vi "open temporary ds opc.vi"(4 "read=f,write=t":bool, 6 "PLC Path and Tag in":T1 {"DataSocket Reference"."OnStatusUpdated" format="%.0x"; "DataSocket Reference"."OnDataUpdated" format="%.0x"}, 8 "error in":errorcluster, 9 "PLC/OPC Path":string, 10 "use opc":bool, 11 "PLC boolean read Tags":T1[](array[typedef]) {"DataSocket Reference"."OnStatusUpdated" format="%.0x"; "DataSocket Reference"."OnDataUpdated" format="%.0x"}) -> (0 "error out":errorcluster, 2 "close ds after io":bool, 3 "PLC Path and Tag out":T1 {"DataSocket Reference"."OnStatusUpdated" format="%.0x"; "DataSocket Reference"."OnDataUpdated" format="%.0x"})   [LabVIEW 2018]
uses:
  05.UserVI's/type defs/plc path and tag.ctl
  <vilib>/Platform/dataskt.llb/DataSocket Reference Type.ctl
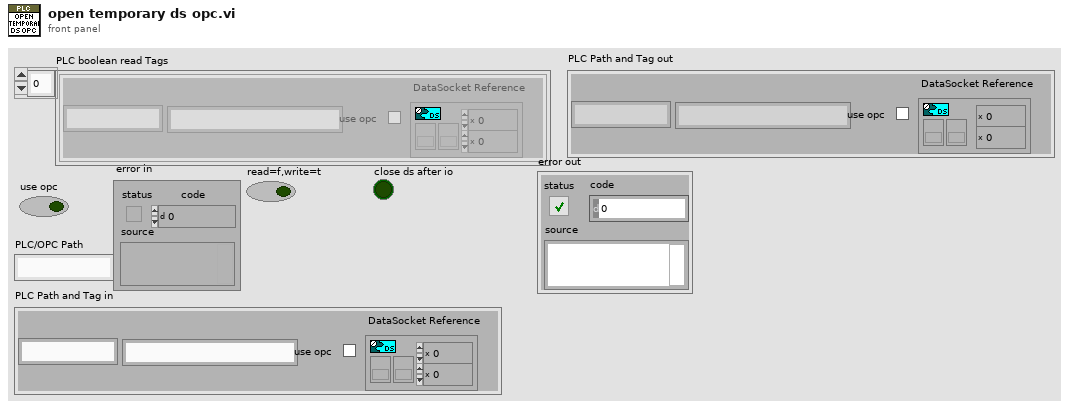
[diagram p1: front panel]
types:
  T1 = typedef "plc path and tag.ctl" = cluster{"Tag Name":string, "Network Path":string, "use opc":bool, "DataSocket Reference":T2}
  T2 = typedef "DataSocket Reference Type.ctl" = cluster{"CWDSLib._DCWDataSocket":refnum<k7>, "CWDSLib._DCWData":refnum<k7>, "OnDataUpdated":u32, "OnStatusUpdated":u32}
  T3 = enum32{"Reserved1", "Reserved2", "Read", "ReadAutoUpdate", "Write", "WriteAutoUpdate"}
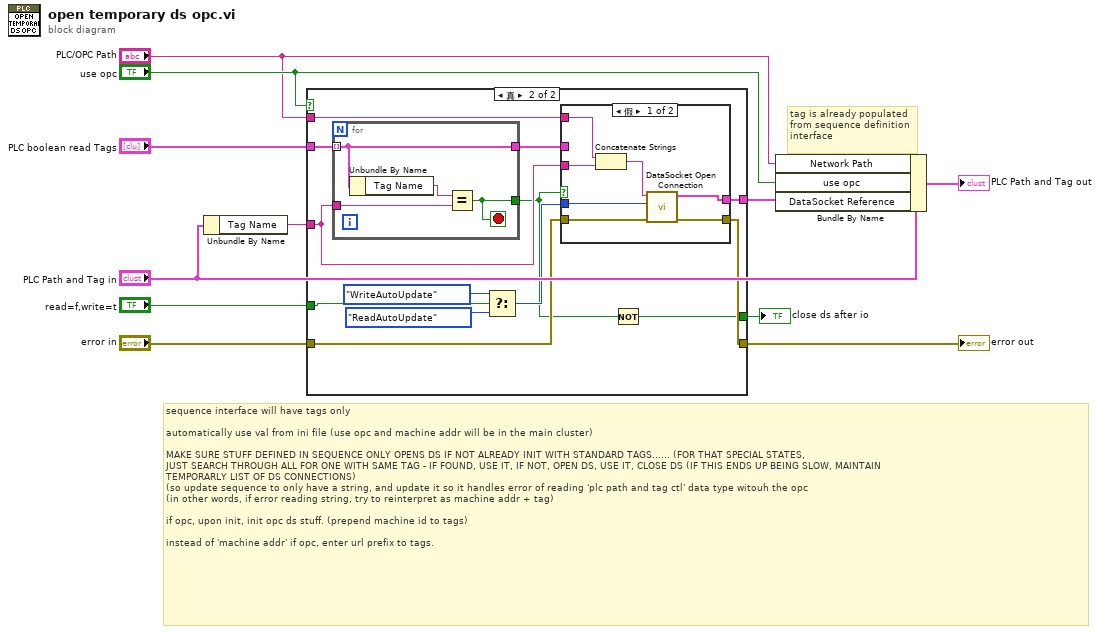
[diagram p0: block diagram]
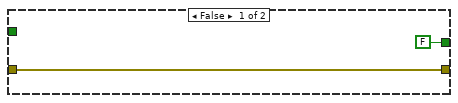
[diagram p2: hidden frame]
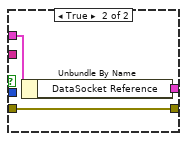
[diagram p3: hidden frame]
diagram:
  # "sequence interface will have tags only\n\nautomatically use val from ini file (use opc and machine addr will be in the main cluster) \n\nMAKE SURE STUFF DEFINED IN SEQUENCE ONLY OPENS DS IF NOT ALREADY INIT WITH STANDARD TAGS...... (FOR THAT SPECIAL STATES,\nJUST SEARCH THROUGH ALL FOR ONE WITH SAME TAG - IF FOUND, USE IT, IF NOT, OPEN DS, USE IT, CLOSE DS (IF THIS ENDS UP BEING SLOW, MAINTAIN\nTEMPORARLY LIST OF DS CONNECTIONS)\n(so update sequence to only have a string, and update it so it handles error of reading 'plc path and tag ctl' data type witouh the opc\n(in other words, if error reading string, try to reinterpret as machine addr + tag)\n\nif opc, upon init, init opc ds stuff. (prepend machine id to tags)\n\ninstead of 'machine addr' if opc, enter url prefix to tags."
  # "tag is already populated from sequence definition interface"
  n1 = Unbundle By Name("PLC Path and Tag in") -> ("Tag Name"=w11:string)
  n2 = case shown="真" "use opc" {
    tunnel: [_ w24] -> w8
    tunnel: "PLC boolean read Tags" -> [_ w26]
    tunnel: w11 -> [_ w20]
    tunnel: "error in" -> [w13 w23]
    tunnel: [w13 w22] -> w4
    tunnel: "PLC/OPC Path" -> [_ w21]
    tunnel: "read=f,write=t" -> [_ w19]
    tunnel: [FALSE w14] -> w1
    frame False {
    }
    frame True {
      n3 = for {
        tunnel: w26 -> [w38] mode=indexing
        tunnel: w20 -> [w39]
        tunnel: [w38] -> w25
        tunnel: [w37] -> w15
        stop <- w37 stop-if-true
        n4 = Unbundle By Name(w38) -> ("Tag Name"=w40:string)
        n5 = Equal?(x=w40, y=w39) -> (x = y?=w37:bool)
      }
      n6 = Select(t=T3."WriteAutoUpdate" ("AccessMode (ReadAutoUpdate)"), s=w19, f=T3."ReadAutoUpdate" ("AccessMode (ReadAutoUpdate)")) -> (s? t:f=w16:T3)
      n7 = case shown="假" w15 {
        tunnel: w25 -> [_ w36]
        tunnel: [w31 w35] -> w24
        tunnel: w23 -> [w33 w34]
        tunnel: [w32 w34] -> w22
        tunnel: w21 -> [w30 _]
        tunnel: w20 -> [w28 _]
        tunnel: w16 -> [w27 _]
        frame False {
          n8 = Concatenate Strings(w30, w28) -> (w29:string)
          n9 = call <vilib>:"DataSocket Open Connection.vi"("error in (no error)"=w33, "AccessMode (ReadAutoUpdate)"=w27, "URL"=w29) -> ("error out"=w32:errorcluster, "DataSocket Reference Out"=w31:T2)  [unwired: 5 in]
        }
        frame True {
          n10 = Unbundle By Name(w36) -> ("DataSocket Reference"=w35:T2)
        }
      }
      n11 = Not(x=w15) -> (.not. x?=w14:bool)
    }
  }
  "error out" <- w4
  "close ds after io" <- w1
  n12 = Bundle By Name(cluster="PLC Path and Tag in", "Network Path"="PLC/OPC Path", "use opc"="use opc", "DataSocket Reference"=w8) -> (→"PLC Path and Tag out":T1)
